vi "Search For Zero.vi"(8 "error in (no error)":errorcluster, 10 "Model in":refnum<class "Model.lvclass">, 11 "Manual State in":refnum<class "Manual State.lvclass">) -> (0 "error out":errorcluster, 2 "Model out":refnum<class "Model.lvclass">, 3 "Manual State out":refnum<class "Manual State.lvclass">)   [LabVIEW 2016, in "Manual State.lvclass"]
uses:
  Manual State.lvclass
  Model/Model/Model.lvclass
  Globals.vi
  Model/Boot Loader/Boot Loader.lvclass
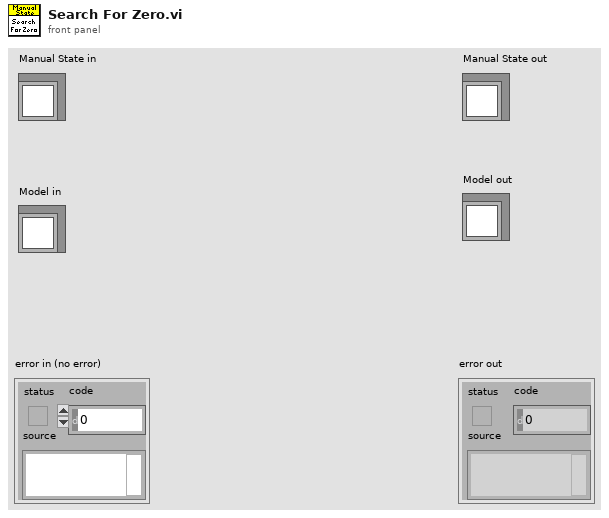
[diagram p1: front panel]
types:
  T1 = typedef "HPMT_Typedefs.lvlib/ActuatorData.ctl" = cluster{"Timestamp":dbl, "Force":dbl, "Encoder Value":i32, "Displacement Sensor 1":dbl, "Displacement Sensor 2":dbl, "Limit Switch CW":bool, "Limit Switch CCW":bool, "Steps Commanded":i32}
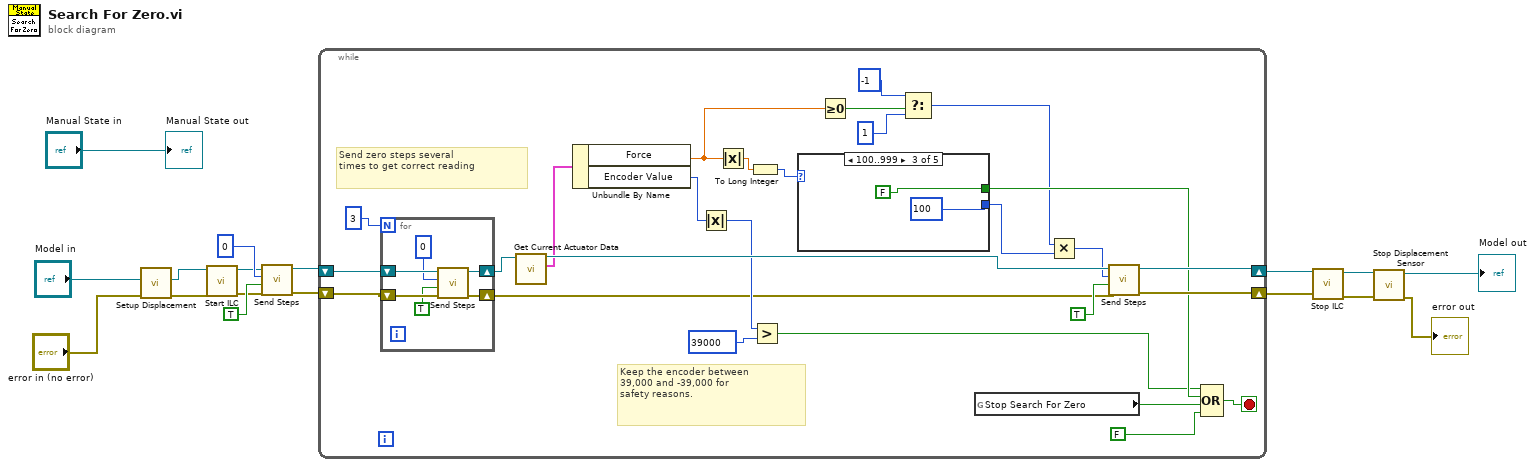
[diagram p0: block diagram]
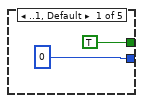
[diagram p2: hidden frame]
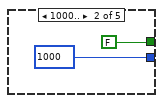
[diagram p3: hidden frame]
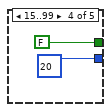
[diagram p4: hidden frame]
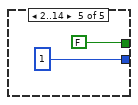
[diagram p5: hidden frame]
diagram:
  n1 = call "Setup Displacement.vi"("error in (no error)"="error in (no error)", "Model in"="Model in") -> ("error out"=w13:errorcluster, "Model out"=w15:refnum<class "Model.lvclass">)  [unwired: 7 in, 1 out]
  n2 = call "Start ILC.vi"("error in (no error)"=w13, "Model in"=w15) -> ("error out"=w4:errorcluster, "Model out"=w3:refnum<class "Model.lvclass">)  [unwired: 8 in]
  n3 = call "Send Steps.vi"("error in (no error)"=w4, "Write Data?"=TRUE, "Command.Steps"=0, "Model in"=w3) -> ("error out"=w1:errorcluster, "Model out"=w2:refnum<class "Model.lvclass">)  [unwired: 6 in]
  n4 = while {
    shift-right: [w43] -> w12
    shift-left: w2 -> [w22]
    shift-right: [w42] -> w9
    shift-left: w1 -> [w20]
    stop <- w37 stop-if-true
    # "Send zero steps several\ntimes to get correct reading"
    # "Keep the encoder between \n39,000 and -39,000 for \nsafety reasons."
    n5 = for {
      N: 3 -> [_]
      shift-right: [w49] -> w21
      shift-left: w22 -> [w50]
      shift-right: [w47] -> w19
      shift-left: w20 -> [w48]
      n6 = call "Send Steps.vi"("error in (no error)"=w48, "Write Data?"=TRUE, "Command.Steps"=0, "Model in"=w50) -> ("error out"=w47:errorcluster, "Model out"=w49:refnum<class "Model.lvclass">)  [unwired: 6 in]
    }
    n7 = call "Get Current Actuator Data.vi"("Model in"=w21) -> ("Actuator Data"=w40:T1, "Model out"=w41:refnum<class "Model.lvclass">)  [unwired: 9 in]
    n8 = Unbundle By Name(w40) -> ("Force"=w23:dbl, "Encoder Value"=w27:i32)
    n9 = Absolute Value(x=w27) -> (abs(x)=w26:i32)
    n10 = Absolute Value(x=w23) -> (abs(x)=w39:dbl)
    n11 = To Long Integer(number=w39) -> (32bit integer=w29:i32)
    n12 = Greater?(x=w26, y=39000) -> (0:w24:bool)
    n13 = case shown="100..999" w29 {
      tunnel: [0 1000 100 20 1] -> w33
      tunnel: [TRUE FALSE FALSE FALSE FALSE] -> w35
      frame ..1, Default {
      }
      frame 1000.. {
      }
      frame 100..999 {
      }
      frame 15..99 {
      }
      frame 2..14 {
      }
    }
    n14 = Greater Or Equal To 0?(x=w23) -> (x >= 0?=w30:bool)
    n15 = Select(t=-1, s=w30, f=1) -> (s? t:f=w28:i32)
    n16 = global read "Globals.vi" "Stop Search For Zero"() -> (w38:bool)
    n17 = Multiply(x=w28, y=w33) -> (x*y=w34:i32)
    n18 = call "Send Steps.vi"("error in (no error)"=w19, "Write Data?"=TRUE, "Command.Steps"=w34, "Model in"=w41) -> ("error out"=w42:errorcluster, "Model out"=w43:refnum<class "Model.lvclass">)  [unwired: 6 in]
    n19 = Compound Arithmetic op=OR(w24, w35, w38, FALSE) -> (w37:bool)
  }
  n20 = call "Stop ILC.vi"("error in (no error)"=w9, "Model in"=w12) -> ("error out"=w8:errorcluster, "Model out"=w11:refnum<class "Model.lvclass">)  [unwired: 8 in]
  n21 = call "Stop Displacement Sensor.vi"("error in (no error)"=w8, "Model in"=w11) -> ("error out"=→"error out":errorcluster, "Model out"=→"Model out":refnum<class "Model.lvclass">)  [unwired: 8 in]
  "Manual State out" <- "Manual State in"
